vi "AssetMgrQueryAssetNodesResponse_Create.vi"(7 "Header":T16, 8 "error in (no error)":errorcluster, 9 "ResponseError":errorcluster, 10 "AssetMgrQueryAssetNodesResponse":T1, 11 "IRoutingSource":T15) -> (0 "error out":errorcluster, 3 "Message":T17)   [LabVIEW 2017]
uses:
  <vilib>/addons/InsightCM/MessageBus/Base/controls/Message.ctl
  <vilib>/addons/InsightCM/MessageBus/Base/controls/MessageHeader.ctl
  <vilib>/addons/InsightCM/MessageBus/Base/controls/KeyValuePair.ctl
  <vilib>/addons/InsightCM/MessageBus/Base/controls/IRoutingSource.ctl
  <vilib>/addons/InsightCM/MessageBus/MessageLibrary/AssetManager/controls/AssetMgrQueryAssetNodesResponseBody.ctl
  <vilib>/addons/InsightCM/MessageBus/Base/controls/AssetNode.ctl
  <vilib>/addons/InsightCM/MessageBus/Base/controls/AssetState.ctl
  <vilib>/addons/InsightCM/MessageBus/Base/controls/AssetNodeSensorGroup.ctl
  <vilib>/addons/InsightCM/MessageBus/Base/controls/WirelessCollectionConfig.ctl
  <vilib>/addons/InsightCM/MessageBus/Base/controls/Condition.ctl
  <vilib>/addons/InsightCM/MessageBus/Base/controls/OperatingState.ctl
  <vilib>/addons/InsightCM/MessageBus/Base/controls/Trigger.ctl
  <vilib>/addons/InsightCM/MessageBus/Base/controls/Metric.ctl
  <vilib>/addons/InsightCM/MessageBus/Base/controls/TrendAlarmRule.ctl
  <vilib>/addons/InsightCM/MessageBus/Base/controls/TrendAlarmLevel.ctl
  <vilib>/addons/InsightCM/MessageBus/Base/controls/AlarmAction.ctl
  <vilib>/addons/InsightCM/MessageBus/Base/controls/AssetNodeReference.ctl
  <vilib>/addons/InsightCM/MessageBus/Base/controls/MessageClassType.ctl
  <vilib>/addons/InsightCM/Utilities/PropertyHelpers/PropertyHelpers.lvlib
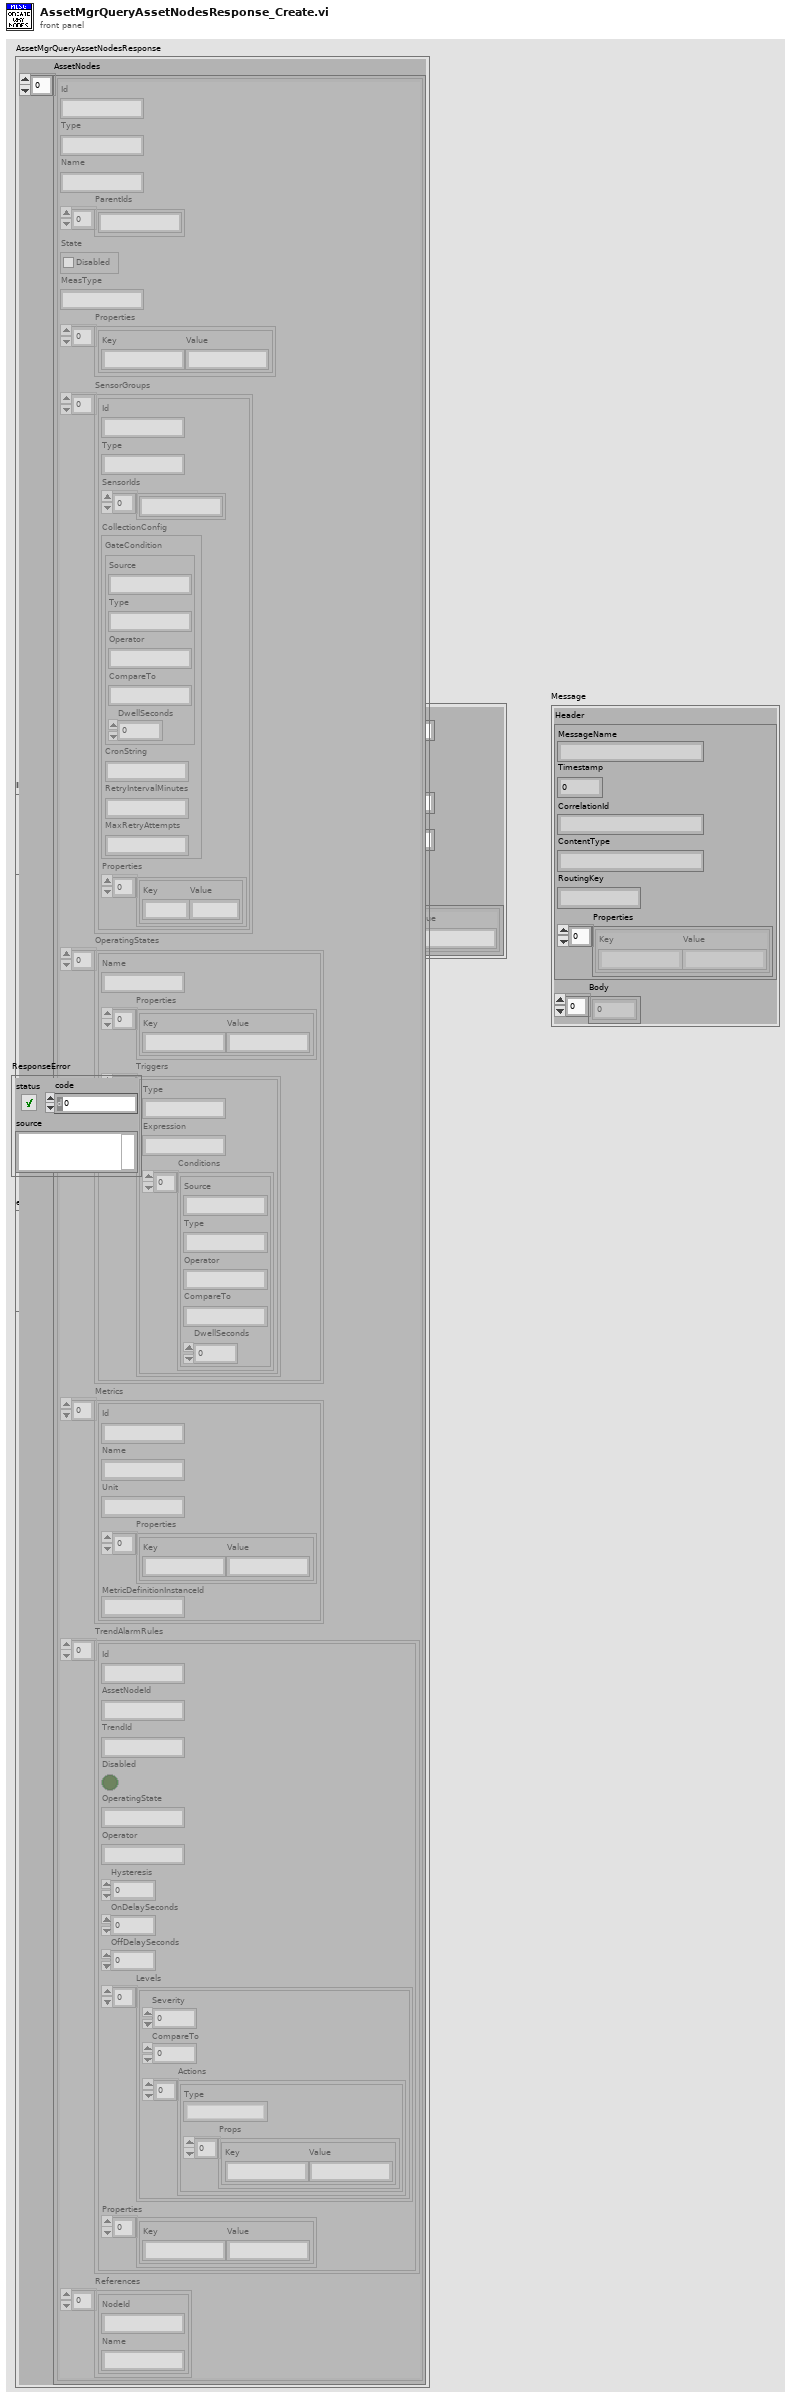
[diagram p1: front panel]
types:
  T1 = typedef "AssetMgrQueryAssetNodesResponseBody.ctl" = cluster{"AssetNodes":T2[]}
  T2 = typedef "AssetNode.ctl" = cluster{"Id":string, "Type":string, "Name":string, "ParentIds":string[], "State":T3, "MeasType":string, "Properties":T4[], "SensorGroups":T5[], "OperatingStates":T8[], "Metrics":T10[], "TrendAlarmRules":T11[], "References":T14[]}
  T3 = typedef "AssetState.ctl" = cluster{"Disabled":bool}
  T4 = typedef "KeyValuePair.ctl" = cluster{"Key":string, "Value":string}
  T5 = typedef "AssetNodeSensorGroup.ctl" = cluster{"Id":string, "Type":string, "SensorIds":string[], "CollectionConfig":T6, "Properties":T4[]}
  T6 = typedef "WirelessCollectionConfig.ctl" = cluster{"GateCondition":T7, "CronString":string, "RetryIntervalMinutes":string, "MaxRetryAttempts":string}
  T7 = typedef "Condition.ctl" = cluster{"Source":string, "Type":string, "Operator":string, "CompareTo":string, "DwellSeconds":dbl}
  T8 = typedef "OperatingState.ctl" = cluster{"Name":string, "Properties":T4[], "Triggers":T9[]}
  T9 = typedef "Trigger.ctl" = cluster{"Type":string, "Expression":string, "Conditions":T7[]}
  T10 = typedef "Metric.ctl" = cluster{"Id":string, "Name":string, "Unit":string, "Properties":T4[], "MetricDefinitionInstanceId":string}
  T11 = typedef "TrendAlarmRule.ctl" = cluster{"Id":string, "AssetNodeId":string, "TrendId":string, "Disabled":bool, "OperatingState":string, "Operator":string, "Hysteresis":dbl, "OnDelaySeconds":dbl, "OffDelaySeconds":dbl, "Levels":T12[], "Properties":T4[]}
  T12 = typedef "TrendAlarmLevel.ctl" = cluster{"Severity":i32, "CompareTo":dbl, "Actions":T13[]}
  T13 = typedef "AlarmAction.ctl" = cluster{"Type":string, "Props":T4[]}
  T14 = typedef "AssetNodeReference.ctl" = cluster{"NodeId":string, "Name":string}
  T15 = typedef "IRoutingSource.ctl" = cluster{"CorrelationId":string, "ReplyTo":string}
  T16 = typedef "MessageHeader.ctl" = cluster{"MessageName":string, "Timestamp":i64, "CorrelationId":string, "ContentType":string, "RoutingKey":string, "Properties":T4[]}
  T17 = typedef "Message.ctl" = cluster{"Header":T16, "Body":u8[]}
  T18 = typedef "MessageClassType.ctl" = enum16{"Request", "Response", "Broadcast", "RoutedMessage"}
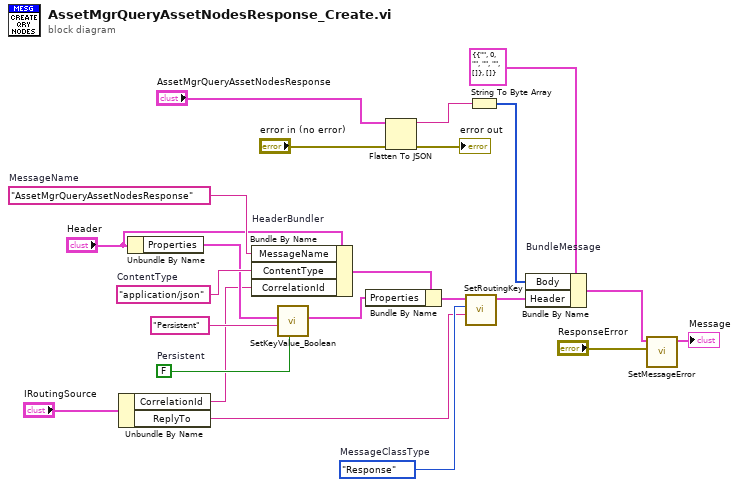
[diagram p0: block diagram]
diagram:
  w19 = MessageClassType."Response"  # MessageClassType
  w14 = FALSE  # Persistent
  w20 = "AssetMgrQueryAssetNodesResponse"  # MessageName
  w17 = "application/json"  # ContentType
  n1 = Unbundle By Name("IRoutingSource") -> ("CorrelationId"=w4:string, "ReplyTo"=w3:string)
  n2 = Unbundle By Name("Header") -> ("Properties"=w16:T4[])
  n3 = Bundle By Name "HeaderBundler"(cluster="Header", "MessageName"=w20, "ContentType"=w17, "CorrelationId"=w4) -> (w11:T16)
  n4 = call <vilib>:"SetKeyValue_Boolean.vi"("value"=w14, "key"="Persistent" ("Key"), "key value pairs"=w16) -> ("key value pairs out"=w10:T4[])  [unwired: 8 in]
  n5 = Bundle By Name(cluster=w11, "Properties"=w10) -> (w12:T16)
  n6 = Flatten To JSON(anything="AssetMgrQueryAssetNodesResponse", error in (no error)="error in (no error)") -> (JSON string=w2:string, 11:→"error out":errorcluster)  [unwired: 1 in]
  n7 = call <vilib>:"SetRoutingKey.vi"("SendTo"=w3, "MessageClassType"=w19, "Message Header in"=w12) -> ("Message Header out"=w13:T16)  [unwired: 8 in]
  n8 = String To Byte Array(string=w2) -> (unsigned byte array=w22:u8[])
  n9 = Bundle By Name "BundleMessage"(cluster=T17 {"Header"={"MessageName"="", "Timestamp"=0, "CorrelationId"="", "ContentType"="", "RoutingKey"="", "Properties"=[]}, "Body"=[]} ("Message"), "Body"=w22, "Header"=w13) -> (w8:T17)
  n10 = call <vilib>:"SetMessageError.vi"("error"="ResponseError", "message in"=w8) -> ("message out"=→"Message":T17)  [unwired: 9 in]
